vi "Read Expected result.vi"(8 "error in (no error)":errorcluster, 11 "[Test Case] File or directory exists in":refnum<class "[Test Case] File or directory exists.lvclass">) -> (0 "error out":errorcluster, 2 "Expected result":bool, 3 "[Test Case] File or directory exists out":refnum<class "[Test Case] File or directory exists.lvclass">)   [LabVIEW 2015, in "Tests.lvlib" / "[Test Case] File or directory exists.lvclass"]
uses:
  [Test Case] File or directory exists.lvclass
  [Test Case] File or directory exists.lvclass/[Test Case] File or directory exists.ctl
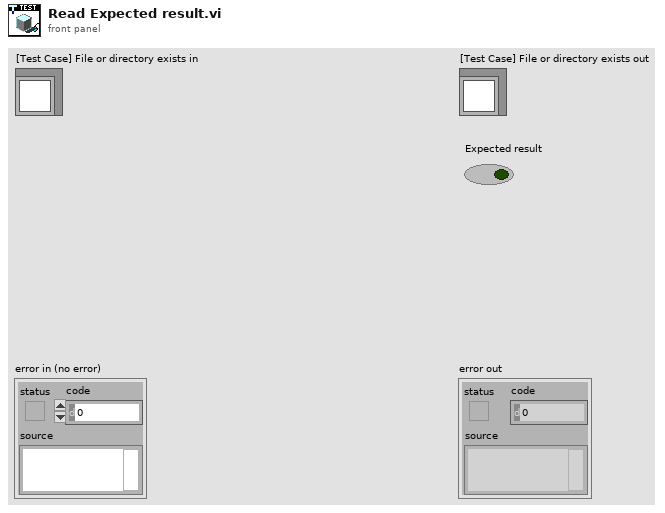
[diagram p1: front panel]
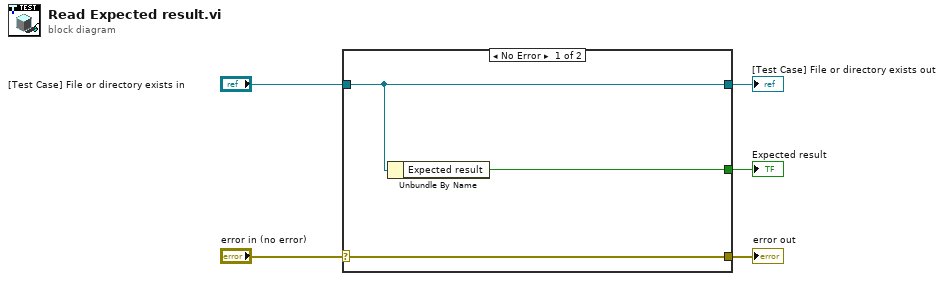
[diagram p0: block diagram]
diagram:
  n1 = case shown="No Error" "error in (no error)" {
    selector: "error in (no error)" -> [w8 w9]
    tunnel: [w8 w9] -> w4
    tunnel: [w7 w10] -> w2
    tunnel: "[Test Case] File or directory exists in" -> [w7 w10]
    tunnel: [w6 _] -> w1
    frame No Error {
      n2 = Unbundle By Name(w7) -> ("Expected result"=w6:bool)
    }
    frame Error {
    }
  }
  "error out" <- w4
  "[Test Case] File or directory exists out" <- w2
  "Expected result" <- w1
